vi "setColumn.vi"(8 "error in (no error)":errorcluster, 11 "reference in":refnum<class "excelFile.lvclass">) -> (0 "error out":errorcluster, 2 "column":i32, 3 "reference out":refnum<class "excelFile.lvclass">)   [LabVIEW 2015, in "excelFile.lvclass"]
uses:
  excelFile.lvclass
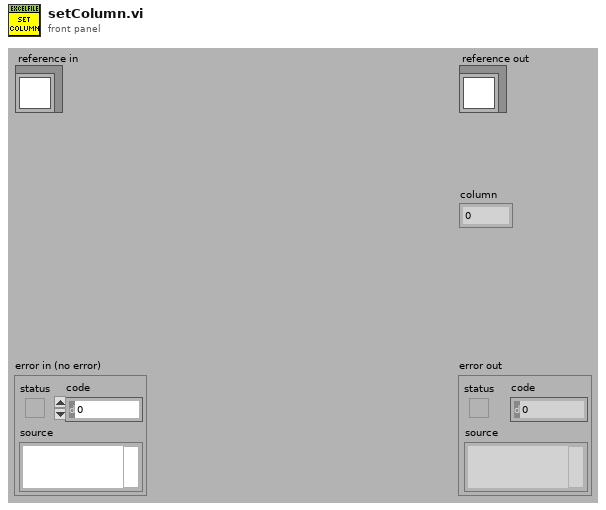
[diagram p1: front panel]
types:
  T1 = typedef "excelFile.lvclass/ObjectAttributesRef.ctl" = refnum<data-value>
  T2 = typedef "excelFile.lvclass/ObjectAttributes.ctl" = cluster{"MyAttribute":dbl, "path":string, "Refnum Excel":cluster{"Excel._Application":refnum<k7>, "Workbooks":refnum<k7>, "Open":refnum<k7>}, "data":string[][][], "fileType":T3, "sheetName":string[]}
  T3 = typedef "excelFile.lvclass/fileType.ctl" = enum16{"database", "CosmedTest"}
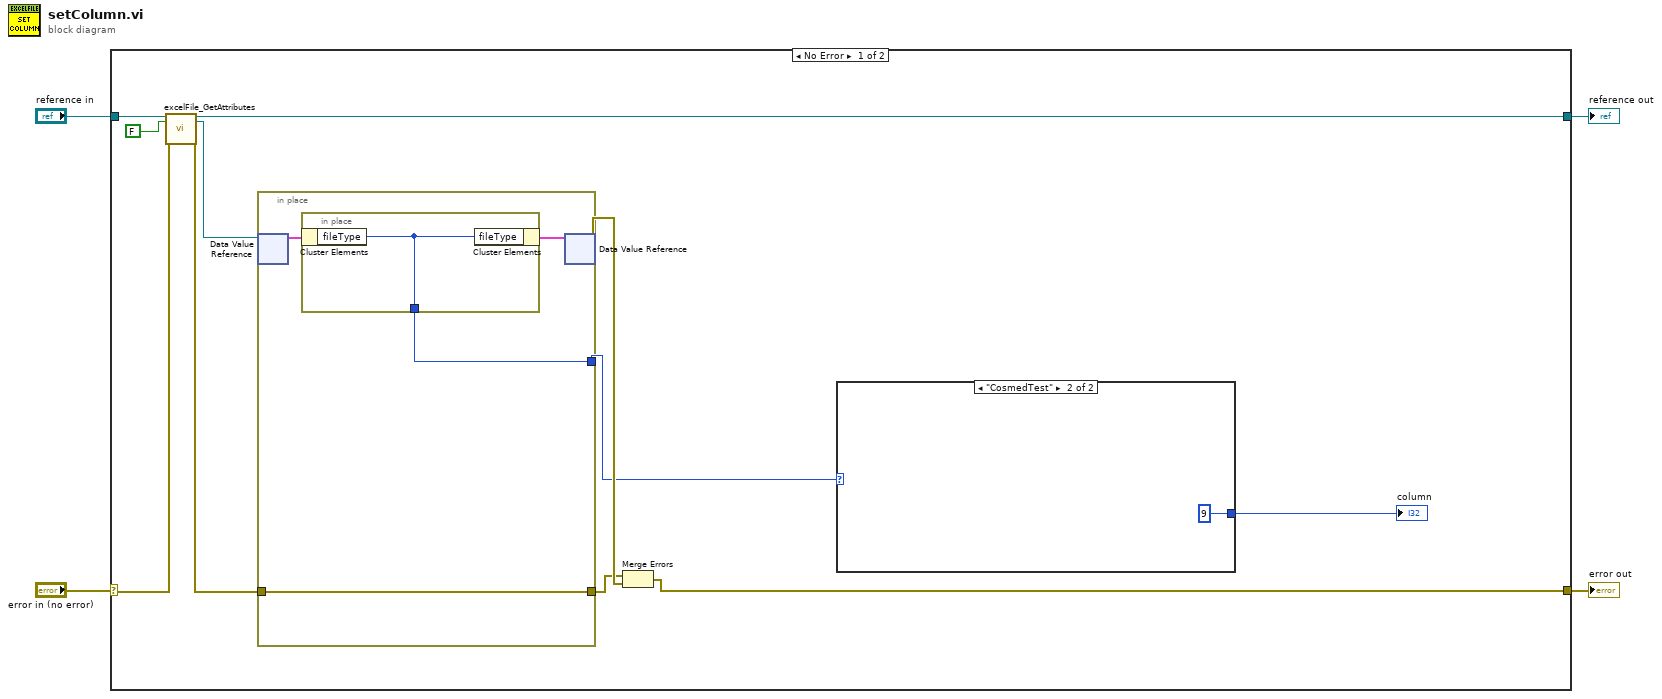
[diagram p0: block diagram]
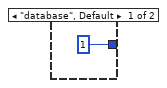
[diagram p2: hidden frame]
diagram:
  n1 = case shown="No Error" "error in (no error)" {
    selector: "error in (no error)" -> [w11 w24]
    tunnel: [w7 w24] -> w3
    tunnel: [w9 w23] -> w1
    tunnel: "reference in" -> [w13 w23]
    frame No Error {
      n2 = call "excelFile_GetAttributes.vi"("reference in"=w13, "return data? (T)"=FALSE, "error in (no error)"=w11) -> ("reference out"=w9:refnum<class "excelFile.lvclass">, "attributes ref"=w8:T1, "error out"=w10:errorcluster)  [unwired: 13 in, 1 out]
      n3 = in-place {
        in-place-border: w10 -> [w19]
        in-place-border: [w19] -> w14
        in-place-border: [w18] -> w5
        n4 = in-place-dvr #1(w8) -> (w20:T2)  [unwired: 1 out]
        n5 = in-place {
          in-place-border: [w22] -> w18
          n6 = in-place-cluster #2(w20) -> ("fileType"=w22:T3)
          n7 = in-place-cluster #2("fileType"=w22) -> (w21:T2)
        }
        n8 = in-place-dvr #1(w21) -> (w15:errorcluster)  [unwired: 1 out]
      }
      n9 = Merge Errors(w14, w15) -> (w7:errorcluster)
      n10 = case shown="\"CosmedTest\"" w5 {
        tunnel: [1 ("Column") 9 ("Column")] -> w6
        frame "database", Default {
        }
        frame "CosmedTest" {
        }
      }
      "column" <- w6
    }
    frame Error {
    }
  }
  "error out" <- w3
  "reference out" <- w1
